vi "ConnectDB.vi"(8 "error in (no error)":errorcluster, 11 "Filename":string="db.mdb") -> (0 "error out":errorcluster, 3 "DB Conn":T1)   [LabVIEW 2020]
uses:
  <vilib>/addons/database/Connection.llb/Conn ObjectReference.ctl
  <vilib>/addons/database/Connection.llb/DB Tools Open Connec (String).vi
  <vilib>/addons/database/NI_Database_API.lvlib
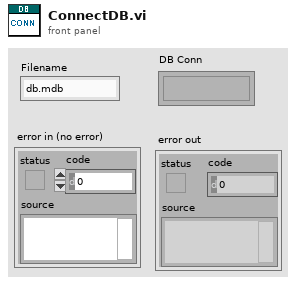
[diagram p1: front panel]
types:
  T1 = typedef "NI_Database_API.lvlib/Conn ObjectReference.ctl" = refnum<k1>
  T2 = enum32{"invalid app kind", "Development System", "Run Time System", "Student Edition", "Embedded LabVIEW", "Evaluation", "Custom"}
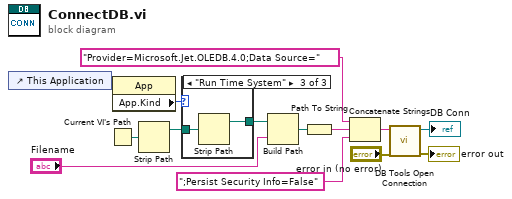
[diagram p0: block diagram]
diagram:
  n1 = control-ref of="This Application"() -> (w8:refnum<vi>)
  n2 = Current VI's Path() -> (path=w9:path)
  n3 = property class="App"(reference=w8) -> ("App.Kind"=w7:T2)  [unwired: 1 in, 2 out]
  n4 = Strip Path(path=w9) -> (stripped path=w6:path)  [unwired: 1 out]
  n5 = case shown="\"Run Time System\"" w7 {
    tunnel: w6 -> [w15 w16 w18]
    tunnel: [w15 w16 w17] -> w5
    frame "invalid app kind", Default {
    }
    frame "Development System" {
    }
    frame "Run Time System" {
      n6 = Strip Path(path=w18) -> (stripped path=w17:path)  [unwired: 1 out]
    }
  }
  n7 = Build Path(base path=w5, name or relative path="Filename") -> (appended path=w13:path)
  n8 = Path To String(path=w13) -> (string=w12:string)
  n9 = Concatenate Strings("Provider=Microsoft.Jet.OLEDB.4.0;Data Source=" ("string"), w12, ";Persist Security Info=False" ("string")) -> (w4:string)
  n10 = call-poly <vilib>:"DB Tools Open Connection.vi"("error in (no error)"="error in (no error)", "connection information"=w4) -> ("error out"=→"error out":errorcluster, "connection reference"=→"DB Conn":T1)  [unwired: 6 in]
